vi "Stop Acquisition.vi"(8 "error in (no error)":errorcluster, 11 "IMAQdx Actor in":refnum<class "IMAQdx Actor.lvclass">) -> (0 "error out":errorcluster, 3 "IMAQdx Actor out":refnum<class "IMAQdx Actor.lvclass">)   [LabVIEW 2020, in "IMAQdx Actor.lvlib" / "IMAQdx Actor.lvclass"]
uses:
  IMAQdx Actor.lvclass
  C:/Users/AlexK/work/LabVIEW Programme/POLARIS CAM Log Abw und E/Submodules/HIJ Vision/Camera Actors/Camera Actor/Camera Actor/Camera Actor.lvclass
  Camera Actor/Camera Actor/Camera Actor.lvclass/Camera Actor.ctl
  Camera Actor/Camera Actor/Operation Mode.ctl
  IMAQdx Actor.lvclass/IMAQdx Actor.ctl
  Camera Actor/Camera Actor/Read Image.vi
  Camera Actor/Camera Actor/Write Camera State.vi
  Camera Actor/Camera Actor/Read Camera State.vi
  Camera Actor/Camera Actor/Camera Actor.lvclass
  <vilib>/vision/driver/NI_Vision_Acquisition_Software.lvlib
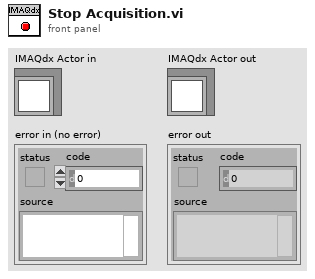
[diagram p1: front panel]
types:
  T1 = typedef "Camera Actor.lvlib/Camera Actor.lvclass/Operation Mode.ctl" = enum16{"Run", "Stop", "Exit", "Error", "Restart"}
  T2 = typedef "IMAQdx.ctl" = refnum<k21>
  T3 = typedef "IMAQ Image.ctl" = refnum<image>
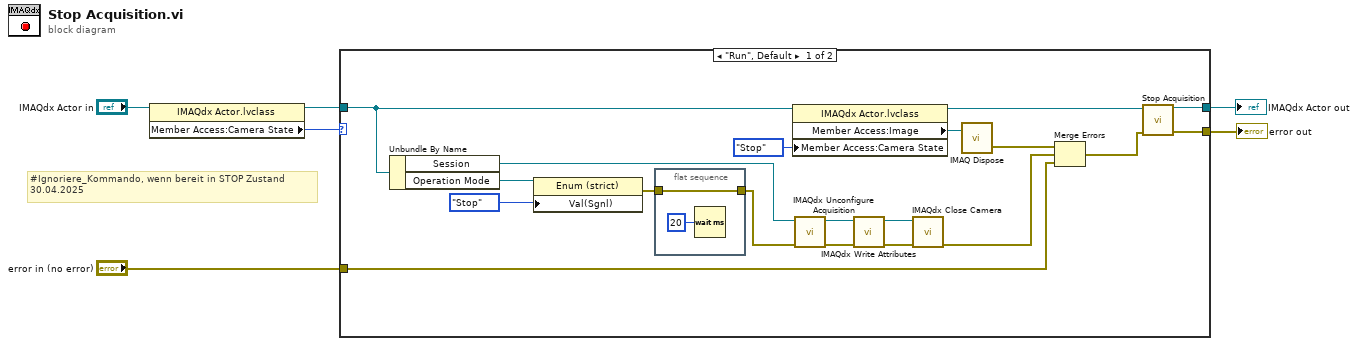
[diagram p0: block diagram]
diagram:
  # "#Ignoriere_Kommando, wenn bereit in STOP Zustand\n30.04.2025"
  n1 = property class="IMAQdx Actor.lvclass"(reference="IMAQdx Actor in") -> (reference out=w4:refnum<class "IMAQdx Actor.lvclass">, "Member Access:Camera State"=w3:T1)  [unwired: 1 in, 1 out]
  n2 = case shown="\"Run\", Default" w3 {
    tunnel: "error in (no error)" -> [w25 w28]
    tunnel: w4 -> [w24 w29]
    tunnel: [w8 w28] -> w2
    tunnel: [w7 w29] -> w1
    frame "Run", Default {
      n3 = Unbundle By Name(w24) -> ("Session"=w14:T2, "Operation Mode"=w15:refnum<vi>)
      n4 = property class="Enum (strict)"(reference=w15, "Val(Sgnl)"=Operation_Mode."Stop" ("Value (Signaling)")) -> (error out=w17:errorcluster)  [unwired: 1 in, 1 out]
      n5 = flat-sequence {
        tunnel: [w26] -> w23
        tunnel: w17 -> [w26]
        frame #0 {
          n6 = Wait (ms)(milliseconds to wait=u32 20) -> ()  [unwired: 1 out]
        }
      }
      n7 = property class="IMAQdx Actor.lvclass"(reference=w24, "Member Access:Camera State"=Operation_Mode."Stop" ("Camera State")) -> (reference out=w9:refnum<class "IMAQdx Actor.lvclass">, "Member Access:Image"=w16:T3)  [unwired: 1 in, 1 out]
      n8 = call <vilib>:"IMAQdx Unconfigure Acquisition.vi"("error in"=w23, "Session In"=w14) -> ("error out"=w13:errorcluster, "Session Out"=w21:T2)  [unwired: 8 out]
      n9 = call <vilib>:"IMAQdx Write Attributes.vi"("error in"=w13, "Session In"=w21) -> ("error out"=w12:errorcluster, "Session Out"=w22:T2)  [unwired: 8 in]
      n10 = call <vilib>:"IMAQdx Close Camera.vi"("error in"=w12, "Session In"=w22) -> ("error out"=w20:errorcluster)  [unwired: 9 out]
      n11 = call "IMAQ Dispose"("Image"=w16) -> ("error out"=w19:errorcluster)  [unwired: 5 in]
      n12 = Merge Errors(w19, w20, w25) -> (w10:errorcluster)
      n13 = call-parent "Stop Acquisition.vi"("error in (no error)"=w10, "Camera in"=w9) -> ("error out"=w8:errorcluster, "Camera out"=w7:refnum<class "IMAQdx Actor.lvclass">)  [unwired: 8 in]
    }
    frame "Stop" {
    }
  }
  "error out" <- w2
  "IMAQdx Actor out" <- w1
